vi "Conveyer Belt Process.vi"(0 "error in":errorcluster) -> ()   [LabVIEW 2012]
uses:
  Conveyer Belt Global Data.vi
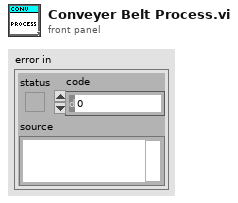
[diagram p1: front panel]
types:
  T1 = cluster{"Horizontal Belt":dbl, "Vertical Belt":dbl, "MS":bool}
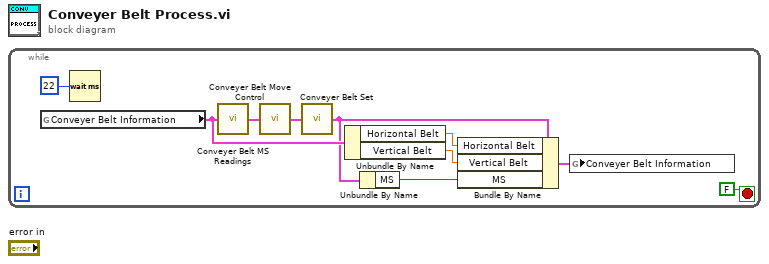
[diagram p0: block diagram]
diagram:
  n1 = while {
    stop <- FALSE stop-if-true
    n2 = global read "Conveyer Belt Global Data.vi" "Conveyer Belt Information"() -> (w6:T1)
    n3 = Wait (ms)(milliseconds to wait=u32 22) -> ()  [unwired: 1 out]
    n4 = call "Conveyer Belt MS Readings.vi"("Conveyer Belt Information In"=w6) -> ("Conveyer Belt Information Out"=w8:T1)
    n5 = call "Conveyer Belt Move Control.vi"("Conveyer Belt Information In"=w8) -> ("Conveyer Belt Information Out"=w7:T1)
    n6 = call "Conveyer Belt Set.vi"("Conveyer Belt Information In"=w7) -> ("Conveyer Belt Information Out"=w4:T1)
    n7 = Unbundle By Name(w6) -> ("Horizontal Belt"=w2:dbl, "Vertical Belt"=w1:dbl)
    n8 = Unbundle By Name(w4) -> ("MS"=w5:bool)
    n9 = Bundle By Name(cluster=w4, "Horizontal Belt"=w2, "Vertical Belt"=w1, "MS"=w5) -> (w3:T1)
    n10 = global write "Conveyer Belt Global Data.vi" "Conveyer Belt Information"(w3) -> ()
  }
